vi "random_average_activity_12.vi"() -> ()   [LabVIEW 2025]
panel:
  in  "Enable":bool=TRUE
  out "RandomSignal":cluster{"number: 0 to 1":dbl, dbl}(graph)
  # "on"
  # "off"
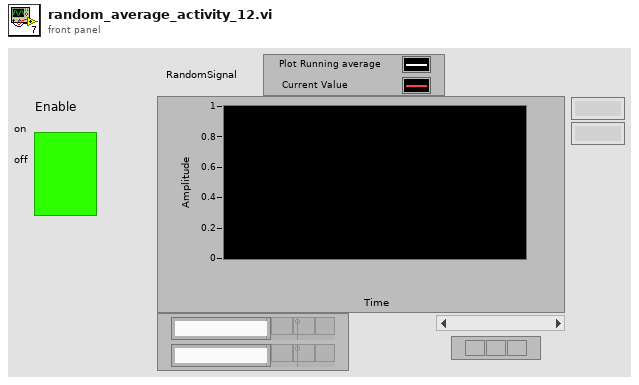
[diagram p1: front panel]
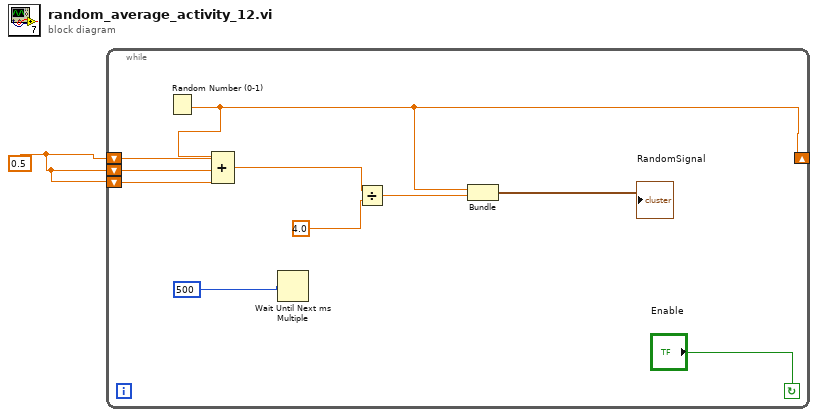
[diagram p0: block diagram]
diagram:
  w1 = 0.5
  n1 = while {
    shift-right: [w4] -> _
    shift-left: w1 -> [w5]
    shift-left: w1 -> [w6]
    shift-left: w1 -> [w7]
    stop <- "Enable" continue-if-true
    n2 = Random Number (0-1)() -> (number: 0 to 1=w4:dbl)
    n3 = Compound Arithmetic op=ADD(w4, w5, w6, w7) -> (w8:dbl)
    n4 = Wait Until Next ms Multiple(millisecond multiple=500) -> ()  [unwired: 1 out]
    n5 = Divide(x=w8, y=4.0) -> (x/y=w3:dbl)
    n6 = Bundle("number: 0 to 1"=w4, w3) -> (→"RandomSignal":cluster{"number: 0 to 1":dbl, dbl})  [unwired: 1 in]
  }
